vi "makeDataJSON.vi"(6 "data array size":i32, 7 "latest notification":T2, 8 "error in":errorcluster, 9 "time stamp (UTC)":dbl, 10 "data cluster array":cluster{"DI2":dbl[]}[](array[cluster]), 11 "StreamCluster_TypeDef":T1={"DAQ"={"ManagmentRate_Hz"=1000, "StreamRate_Hz"=10, "StreamRate_ms"=0, "ManagmentRate_ms"=1000, "refDesArray"=[]}, "Modules"=[]}) -> (0 "error out":errorcluster, 3 "JSON Package":string)   [LabVIEW 2024]
uses:
  Control/Control Data Constant.ctl
  Control/StreamCluster_TypeDef.ctl
  38111faf-85f9-4c31-b2be-400358d47020.vi
  d23956e0-d9d2-468d-8138-a83dba552ec3.vi
  6f7d2803-0a66-4d35-ba1c-fa345de558b7.vi
  5116178f-0dfb-48c9-9625-9b9158091d86.vi
  3b1a1b6f-152a-46d7-9bcd-f8e992418117.vi
  <vilib>/JDP Science/JSONtext/Variant to JSON Text.vi
  <vilib>/JDP Science/JSONtext/Get all Object Items.vi
  <vilib>/JDP Science/JSONtext/Set Multiple Object Items.vi
  <vilib>/JDP Science/JSONtext/LVClass Serializer/JSONtext LVClass Serializer.lvclass
  <vilib>/JDP Science/JSONtext/JSONtext.lvlib
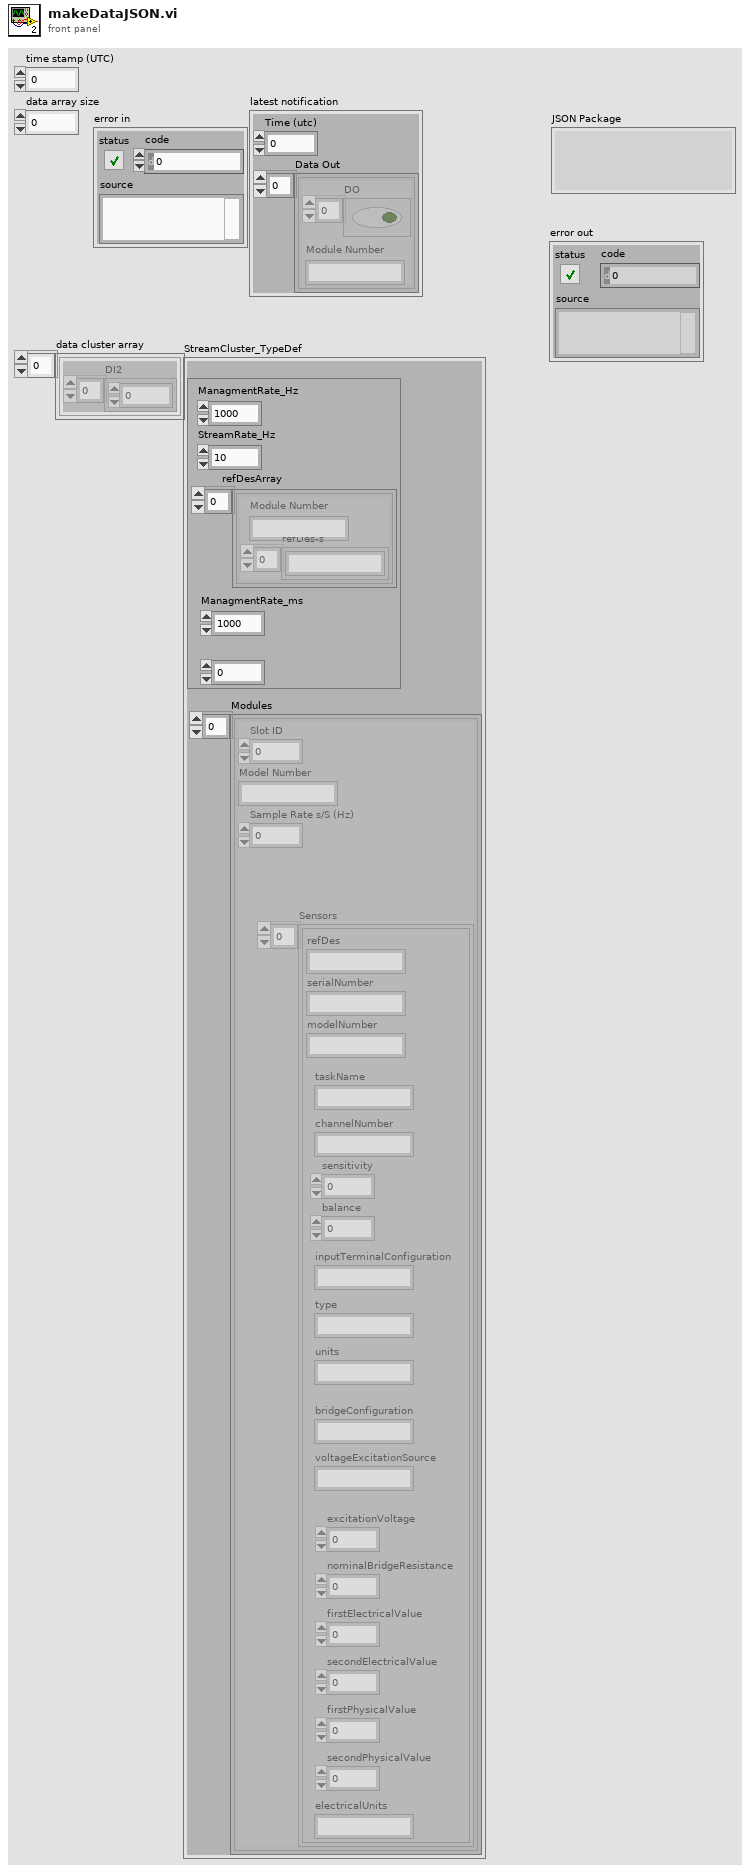
[diagram p1: front panel]
types:
  T1 = typedef "StreamCluster_TypeDef.ctl" = cluster{"DAQ":cluster{"ManagmentRate_Hz":i32, "StreamRate_Hz":i32, "StreamRate_ms":i32, "ManagmentRate_ms":i32, "refDesArray":cluster{"refDes-s":string[], "Module Number":string}[]}, "Modules":cluster{"Slot ID":i32, "Model Number":string, "Sample Rate s/S (Hz)":dbl, "Sensors":cluster{"refDes":string, "serialNumber":string, "modelNumber":string, "units":string, "balance":dbl, "sensitivity":dbl, "type":string, "inputTerminalConfiguration":string, "channelNumber":string, "taskName":string, "bridgeConfiguration":string, "excitationVoltage":dbl, "voltageExcitationSource":string, "nominalBridgeResistance":dbl, "firstElectricalValue":dbl, "secondElectricalValue":dbl, "firstPhysicalValue":dbl, "secondPhysicalValue":dbl, "electricalUnits":string}[]}[]}
  T2 = typedef "Control Data Constant.ctl" = cluster{"Time (utc)":ext, "Data Out":cluster{"DO":bool[], "Module Number":string}[]}
  T3 = cluster{"refDes-s":string[], "Module Number":string}[]
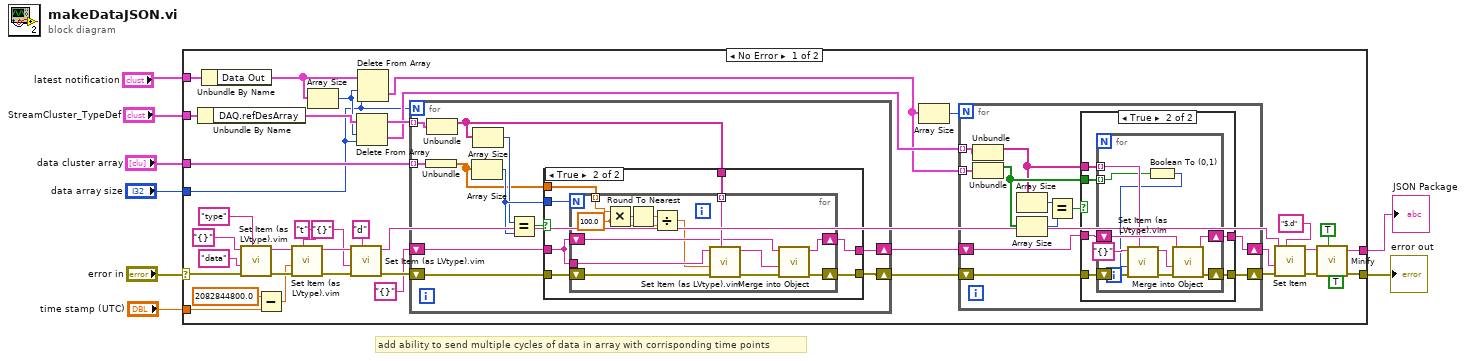
[diagram p0: block diagram]
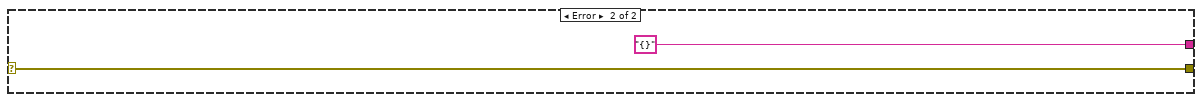
[diagram p4: hidden frame]
diagram:
  # "add ability to send multiple cycles of data in array with corrisponding time points"
  n1 = case shown="No Error" "error in" {
    selector: "error in" -> [w35 w111]
    tunnel: [w27 w111] -> w7
    tunnel: [w26 "{}" ("<JSON>")] -> w6
    tunnel: "time stamp (UTC)" -> [w46 _]
    tunnel: "data cluster array" -> [w23 _]
    tunnel: "latest notification" -> [w20 _]
    tunnel: "StreamCluster_TypeDef" -> [w14 _]
    tunnel: "data array size" -> [w10 _]
    frame No Error {
      n2 = Unbundle By Name(w14) -> ("DAQ.refDesArray"=w13:T3)
      n3 = Unbundle By Name(w20) -> ("Data Out"=w12:cluster{"DO":bool[], "Module Number":string}[])
      n4 = call "Set Item (as LVtype).vim"("$Path or Item Name"="type", "error in (no error)"=w35, "Anything"="data" ("JSON"), "JSON"="{}") -> ("error out"=w42:errorcluster, "<JSON>"=w43:string)  [unwired: 4 in, 1 out]
      n5 = Subtract(x=2082844800.0, y=w46) -> (x-y=w34:dbl)
      n6 = call "Set Item (as LVtype).vim"("$Path or Item Name"="t", "error in (no error)"=w42, "Anything"=w34, "JSON"=w43) -> ("error out"=w44:errorcluster, "<JSON>"=w45:string)  [unwired: 4 in, 1 out]
      n7 = Array Size(array=w12) -> (size(s)=w11:i32)
      n8 = call "Set Item (as LVtype).vim"("$Path or Item Name"="d", "error in (no error)"=w44, "Anything"="{}" ("JSON"), "JSON"=w45) -> ("error out"=w33:errorcluster, "<JSON>"=w25:string)  [unwired: 4 in, 1 out]
      n9 = Delete From Array(array=w13, length=w11, index=w10) -> (deleted portion=w15:T3, array with subset deleted=w16:T3)
      n10 = Delete From Array(array=w12, length=w11, index=w10) -> (deleted portion=w9:cluster{"DO":bool[], "Module Number":string}[])  [unwired: 1 out]
      n11 = for {
        N: w10 -> [_]
        tunnel: w16 -> [w80] mode=indexing
        shift-right: [w85] -> w22
        shift-left: w33 -> [w77]
        tunnel: w23 -> [w82] mode=indexing
        shift-right: [w87] -> w21
        shift-left: "{}" ("JSON") -> [w78]
        n12 = Unbundle(w82) -> ("DI2"=w81:dbl[])
        n13 = Unbundle(w80) -> ("refDes-s"=w79:string[])  [unwired: 1 out]
        n14 = Array Size(array=w81) -> (size(s)=w84:i32)
        n15 = Array Size(array=w79) -> (size(s)=w83:i32)
        n16 = Equal?(x=w83, y=w84) -> (x = y?=w86:bool)
        n17 = case shown="True" w86 {
          tunnel: w77 -> [w89 w96]
          tunnel: [w89 w90] -> w85
          tunnel: w78 -> [w88 w92]
          tunnel: [w88 w91] -> w87
          tunnel: w79 -> [_ w95]
          tunnel: w84 -> [_ w94]
          tunnel: w81 -> [_ w93]
          frame False {
          }
          frame True {
            n18 = for {
              N: w94 -> [_]
              shift-right: [w103] -> w91
              shift-left: w92 -> [w104]
              tunnel: w95 -> [w108] mode=indexing
              tunnel: w93 -> [w98] mode=indexing
              tunnel: w92 -> [w107]
              shift-right: [w102] -> w90
              shift-left: w96 -> [w109]
              w99 = 100.0 ("y")
              n19 = Multiply(x=w98, y=w99) -> (x*y=w100:dbl)
              n20 = Round To Nearest(number=w100) -> (nearest integer value=w101:dbl)
              n21 = Divide(x=w101, y=w99) -> (x/y=w97:dbl)
              n22 = call "Set Item (as LVtype).vim"("$Path or Item Name"=w108, "error in (no error)"=w109, "Anything"=w97, "JSON"=w107) -> ("error out"=w106:errorcluster, "<JSON>"=w105:string)  [unwired: 4 in, 1 out]
              n23 = call <vilib>:"Merge into Object.vi"("error in (no error)"=w106, "JSON Object to Merge"=w105, "JSON"=w104) -> ("error out"=w102:errorcluster, "<JSON>"=w103:string)  [unwired: 6 in]
            }
          }
        }
      }
      n24 = Array Size(array=w9) -> (size(s)=w19:i32)
      n25 = for {
        N: w19 -> [_]
        shift-right: [w51] -> w17
        shift-left: w22 -> [w50]
        shift-right: [w53] -> w18
        shift-left: w21 -> [w52]
        tunnel: w9 -> [w57] mode=indexing
        tunnel: w15 -> [w58] mode=indexing
        n26 = Unbundle(w58) -> ("refDes-s"=w48:string[])  [unwired: 1 out]
        n27 = Unbundle(w57) -> ("DO"=w49:bool[])  [unwired: 1 out]
        n28 = Array Size(array=w48) -> (size(s)=w54:i32)
        n29 = Array Size(array=w49) -> (size(s)=w55:i32)
        n30 = Equal?(x=w54, y=w55) -> (x = y?=w56:bool)
        n31 = case shown="True" w56 {
          tunnel: [w60 w63] -> w53
          tunnel: w52 -> [w60 w64]
          tunnel: [w59 w65] -> w51
          tunnel: w50 -> [w59 w66]
          tunnel: w49 -> [_ w62]
          tunnel: w48 -> [_ w61]
          frame False {
          }
          frame True {
            n32 = for {
              shift-right: [w69] -> w65
              shift-left: w66 -> [w76]
              shift-right: [w72] -> w63
              shift-left: w64 -> [w73]
              tunnel: w62 -> [w68] mode=indexing
              tunnel: w61 -> [w71] mode=indexing
              n33 = Boolean To (0,1)(Boolean=w68) -> (0, 1=w67:i16)
              n34 = call "Set Item (as LVtype).vim"("$Path or Item Name"=w71, "error in (no error)"=w76, "Anything"=w67, "JSON"="{}") -> ("error out"=w75:errorcluster, "<JSON>"=w74:string)  [unwired: 4 in, 1 out]
              n35 = call <vilib>:"Merge into Object.vi"("error in (no error)"=w75, "JSON Object to Merge"=w74, "JSON"=w73) -> ("error out"=w69:errorcluster, "<JSON>"=w72:string)  [unwired: 6 in]
            }
          }
        }
      }
      n36 = call <vilib>:"Set Item.vi"("$Path or Item Name"="$.d", "error in (no error)"=w17, "JSON to Insert"=w18, "JSON"=w25) -> ("error out"=w31:errorcluster, "<JSON>"=w32:string)  [unwired: 4 in, 1 out]
      n37 = call <vilib>:"Minify.vi"("Disable LabVIEW Extensions"=TRUE, "Drop Object Items that are null"=TRUE, "error in (no error)"=w31, "JSON"=w32) -> ("error out"=w27:errorcluster, "<JSON>"=w26:string)  [unwired: 5 in, 1 out]
    }
    frame Error {
    }
  }
  "error out" <- w7
  "JSON Package" <- w6
